vi "DAQ_UI.TestLauncher.vi"() -> ()   [LabVIEW 2020, in "DAQ_UI.lvclass"]
doc: "JKI State Machine Objects (SMO) 1.0.0.5\nJKI - JKI\nCopyright (c) 2016, JKI"
uses:
  DAQ_UI.lvclass
  C:/Program Files (x86)/National Instruments/LabVIEW 2020/vi.lib/JKI/JKI SMO/SMO/SMO.lvclass
  C:/Program Files (x86)/National Instruments/LabVIEW 2020/vi.lib/JKI/JKI SMO/SMO.UI/SMO.UI.lvclass
  <vilib>/JKI/JKI SMO/SMO/SMO.lvclass/SMO.ctl
  <vilib>/JKI/JKI SMO/SMO.UI/SMO.UI.lvclass/SMO.UI.ctl
  <vilib>/JKI/JKI SMO/SMO/Typedefs/SMOState --Enum.ctl
  <vilib>/JKI/JKI SMO/SMO/Private/ReftoDVR--SMO.vi
  <vilib>/JKI/JKI SMO/SMO.UI/SMO.UI.ReftoDVR.vi
  <vilib>/JKI/JKI SMO/SMO/SMO.lvclass
  <vilib>/JKI/JKI SMO/SMO.UI/SMO.UI.lvclass
  D:/BingoGithub/DAQ_V000.00/DAQ_UI/DAQ_UI.lvclass
panel:
  in  "ShowUI":bool
  in  "Send":bool
  in  "Data":string
  out "error out":errorcluster
  in  "Stop":bool
  # "SMO UI Test Launcher"
  # "For instructions on how to use the JKI State Machine Objects, examples and video tutorials, visit:\nhttp://jki.net/state-machine-objects/\n\nJKI State Machine Objects™\nhttp://jki.net/state-machine-objects/\nCopyright (C) 2005-2015, JKI <info@jki.net>\nALL RIGHTS RESERVED"
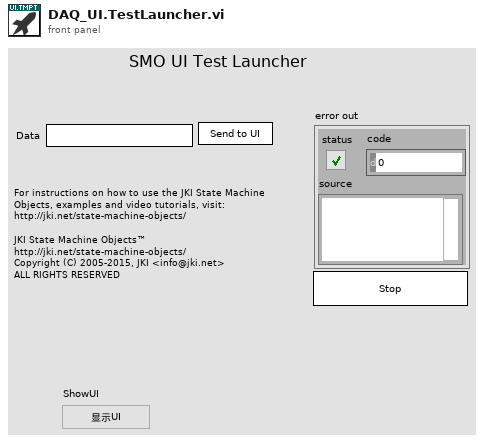
[diagram p1: front panel]
types:
  T1 = typedef "DAQ_UI.lvclass/PublicEvents--Cluster.ctl" = cluster{"Data Changed":refnum<user-event>}
  T2 = typedef "SMO.lvclass/Public Events.ctl" = cluster{"Error":refnum<user-event>, "State":refnum<user-event>, "Reserve State":refnum<user-event>}
  T3 = typedef "SMO.UI.lvclass/PublicEvents--Cluster.ctl" = cluster{"UI Hidden":refnum<user-event>, "UI State":refnum<user-event>}
  T4 = typedef "SMO.lvclass/SMOState --Enum.ctl" = enum16{"unknown", "Created", "Started", "Stopped"}
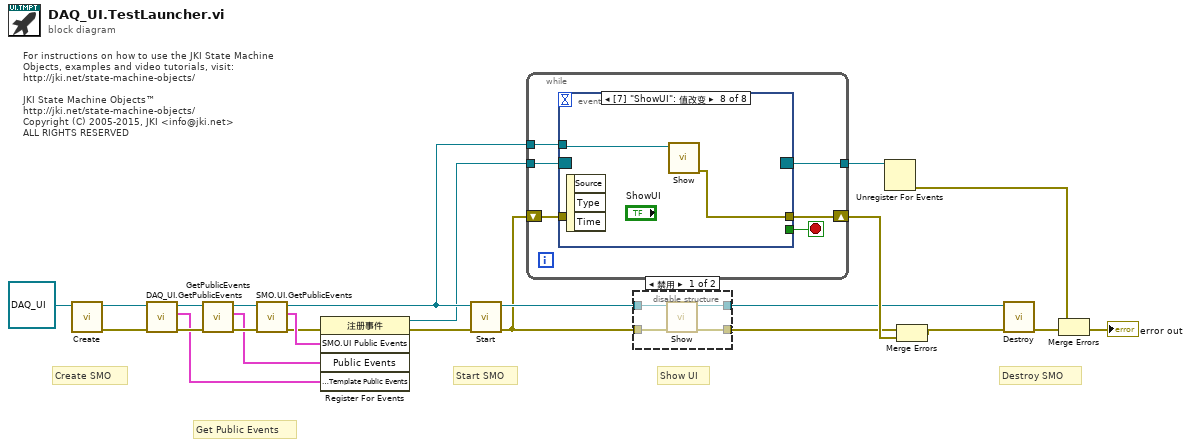
[diagram p0: block diagram]
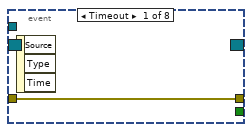
[diagram p3: hidden frame]
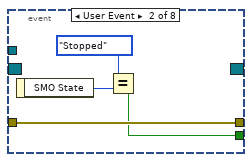
[diagram p4: hidden frame]
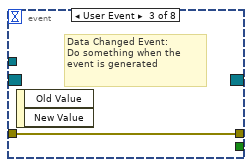
[diagram p5: hidden frame]
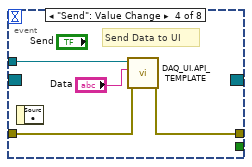
[diagram p6: hidden frame]
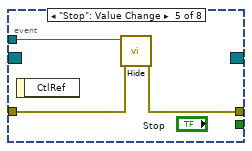
[diagram p7: hidden frame]
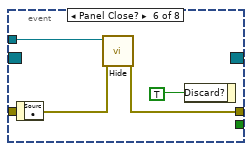
[diagram p8: hidden frame]
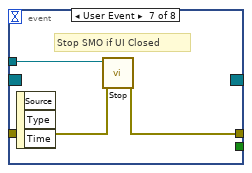
[diagram p9: hidden frame]
diagram:
  # "Get Public Events"
  # "Show UI"
  # "For instructions on how to use the JKI State Machine Objects, examples and video tutorials, visit:\nhttp://jki.net/state-machine-objects/\n\nJKI State Machine Objects™\nhttp://jki.net/state-machine-objects/\nCopyright (C) 2005-2015, JKI <info@jki.net>\nALL RIGHTS RESERVED"
  # "Start SMO"
  # "Destroy SMO"
  # "Create SMO"
  n1 = call <vilib>:"Create.vi"("SMO"=refnum<class "DAQ_UI.lvclass"> refnum ("SMO.Template.lvclass")) -> ("error out"=w6:errorcluster, "SMO out"=w8:refnum<class "DAQ_UI.lvclass">)  [unwired: 8 in, 1 out]
  n2 = call "DAQ_UI.GetPublicEvents.vi"("error in (no error)"=w6, "DAQ_UI"=w8) -> ("error out"=w5:errorcluster, "SMO.Template Public Events"=w4:T1, "DAQ_UI out"=w7:refnum<class "DAQ_UI.lvclass">)  [unwired: 7 in]
  n3 = call <vilib>:"GetPublicEvents.vi"("error in (no error)"=w5, "SMO"=w7) -> ("error out"=w10:errorcluster, "Public Events"=w9:T2, "SMO out"=w11:refnum<class "DAQ_UI.lvclass">)  [unwired: 7 in]
  n4 = call <vilib>:"SMO.UI.GetPublicEvents.vi"("error in (no error)"=w10, "SMO.UI"=w11) -> ("error out"=w14:errorcluster, "SMO.UI Public Events"=w15:T3, "SMO.UI out"=w13:refnum<class "DAQ_UI.lvclass">)  [unwired: 7 in]
  n5 = register-events(error in=w14, w15, w9, w4) -> (reference out=w3:refnum<event-registration>, error out=w12:errorcluster)  [unwired: 1 in]
  n6 = call <vilib>:"Start.vi"("error in (no error)"=w12, "SMO"=w13) -> ("error out"=w17:errorcluster, "SMO out"=w18:refnum<class "DAQ_UI.lvclass">)  [unwired: 8 in]
  n7 = while {
    shift-right: [w29] -> w23
    shift-left: w17 -> [w28]
    tunnel: w3 -> [w27]
    tunnel: [w26] -> w24
    tunnel: w13 -> [w25]
    stop <- w30 stop-if-true
    n8 = event shown="[7] \"ShowUI\": 值改变" {
      selector: w27 -> [_ _ _ _ _ _ _ _]
      dyn-events: [_ _ _ _ _ _ _ _] -> w26
      timeout: _ -> [_ _ _ _ _ _ _ _]
      tunnel: [_ w32 _ _ _ _ _ _] -> w30
      tunnel: w25 -> [_ _ _ w40 w43 w46 w50 w52]
      tunnel: [w31 w35 w36 w37 w41 w44 w49 w51] -> w29
      tunnel: w28 -> [w31 w35 w36 w38 w42 w45 w48 _]
      event Timeout {
        n9 = event-data() -> ()  [unwired: 1 in, 3 out]
      }
      event User Event {
        n10 = event-data() -> ("SMO State"=w34:T4)  [unwired: 1 in]
        n11 = Equal?(x=SMOState_--Enum."Stopped", y=w34) -> (x = y?=w32:bool)
      }
      event User Event {
        # "Data Changed Event:\nDo something when the\nevent is generated"
        n12 = event-data() -> ()  [unwired: 1 in, 2 out]
      }
      event "Send": Value Change {
        # "Send Data to UI"
        n13 = event-data() -> ()  [unwired: 1 in, 1 out]
        n14 = call "DAQ_UI.API_TEMPLATE.vi"("error in (no error)"=w38, "myData"="Data", "DAQ_UI"=w40) -> ("error out"=w37:errorcluster)  [unwired: 6 in, 2 out]
      }
      event "Stop": Value Change {
        n15 = event-data() -> ()  [unwired: 1 in, 1 out]
        n16 = call <vilib>:"Hide.vi"("error in (no error)"=w42, "SMO.UI"=w43) -> ("error out"=w41:errorcluster)  [unwired: 8 in, 1 out]
      }
      event Panel Close? {
        n17 = event-data() -> ()  [unwired: 1 in, 1 out]
        n18 = call <vilib>:"Hide.vi"("error in (no error)"=w45, "SMO.UI"=w46) -> ("error out"=w44:errorcluster)  [unwired: 8 in, 1 out]
        n19 = event-data("Discard?"=TRUE ("OK")) -> ()  [unwired: 1 in, 1 out]
      }
      event User Event {
        # "Stop SMO if UI Closed"
        n20 = event-data() -> ()  [unwired: 1 in, 3 out]
        n21 = call <vilib>:"Stop.vi"("error in (no error)"=w48, "SMO"=w50) -> ("error out"=w49:errorcluster)  [unwired: 8 in, 1 out]
      }
      event "ShowUI": Value Change {
        n22 = event-data() -> ()  [unwired: 1 in, 3 out]
        n23 = call <vilib>:"Show.vi"("SMO.UI"=w52) -> ("error out"=w51:errorcluster)  [unwired: 9 in, 1 out]
      }
    }
  }
  n24 = disable-structure shown="禁用" {
    disable-tunnel: w18 -> [w56 w58]
    disable-tunnel: w17 -> [w55 w57]
    disable-tunnel: [w54 w57] -> w16
    disable-tunnel: [w53 w58] -> w1
    frame Disabled {
      n25 = call <vilib>:"Show.vi"("error in (no error)"=w55, "SMO.UI"=w56) -> ("error out"=w54:errorcluster, "SMO.UI out"=w53:refnum<class "DAQ_UI.lvclass">)  [unwired: 8 in]
    }
    frame Enabled {
    }
  }
  n26 = Unregister For Events(event registration refnum=w24) -> (error out=w22:errorcluster)  [unwired: 1 in]
  n27 = Merge Errors(w16, w23) -> (w2:errorcluster)
  n28 = call <vilib>:"Destroy.vi"("error in (no error)"=w2, "SMO"=w1) -> ("error out"=w20:errorcluster)  [unwired: 9 in]
  n29 = Merge Errors(w22, w20) -> (→"error out":errorcluster)
